vi "RT Main.vi"() -> ()   [LabVIEW 2021]
panel:
  out "current time":timestamp
  in  "stop":bool
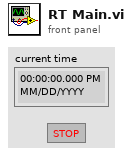
[diagram p1: front panel]
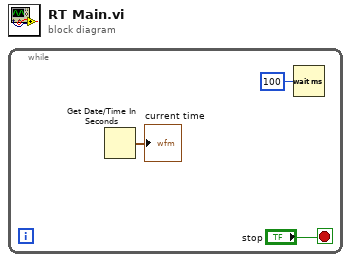
[diagram p0: block diagram]
diagram:
  n1 = while {
    stop <- "stop" stop-if-true
    n2 = Get Date/Time In Seconds() -> (seconds since 1Jan1904=→"current time":timestamp)
    n3 = Wait (ms)(milliseconds to wait=u32 100) -> ()  [unwired: 1 out]
  }
